vi "Com_SECS Equipment _Data Message Tree.vi"(8 "error in":errorcluster, 10 "SECS Packet":T1, 11 "Tree Refnum":refnum<vi>) -> (0 "error out":errorcluster)   [LabVIEW 2016]
uses:
  Data Def/Com_SECS Equipment _SECS Packet.ctl
  Data Def/Com_SECS Equipment _Message Type.ctl
  Data Def/Com_SECS Equipment _Protocol Type.ctl
  Data Def/Com_SECS Equipment _Stream Type.ctl
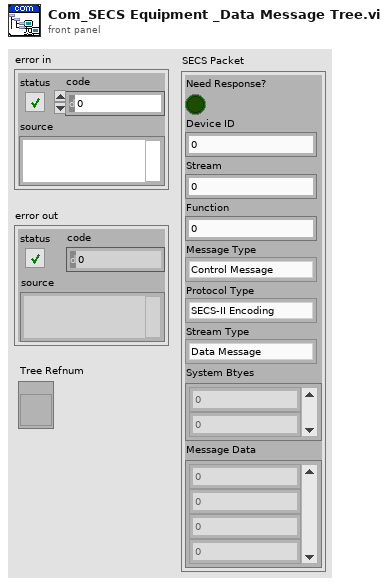
[diagram p1: front panel]
types:
  T1 = typedef "Com_SECS Equipment _SECS Packet.ctl" = cluster{"Need Response?":bool, "Device ID":u16, "Stream":u8, "Function":u8, "Message Type":T2, "Protocol Type":T3, "Stream Type":T4, "System Btyes":u8[], "Message Data":u8[]}
  T2 = typedef "Com_SECS Equipment _Message Type.ctl" = enum16{"Control Message", "Data Message"}
  T3 = typedef "Com_SECS Equipment _Protocol Type.ctl" = enum16{"SECS-II Encoding", "Reserved"}
  T4 = typedef "Com_SECS Equipment _Stream Type.ctl" = enum16{"Data Message", "Select.req", "Select.rsp", "Deselect.req", "Deselect.rsp", "Linktest.req", "Linktest.rsp", "Reject.req", "Separate.req", "Reserve"}
  T5 = typedef "Com_SECS Equipment _Message Data.ctl" = cluster{"Index":i32, "Data Item Format":T6, "Format Code":T7, "Parent Index":i32, "Child Index":i32[], "Data":variant}
  T6 = typedef "Com_SECS Equipment _Data Item Format.ctl" = enum16{"Data Type", "Value"}
  T7 = typedef "Com_SECS Equipment _Format Code.ctl" = enum16{"L", "A", "B", "Boolean", "J", "I1", "I2", "I4", "I8", "U1", "U2", "U4", "U8", "F4", "F8", "Char"}
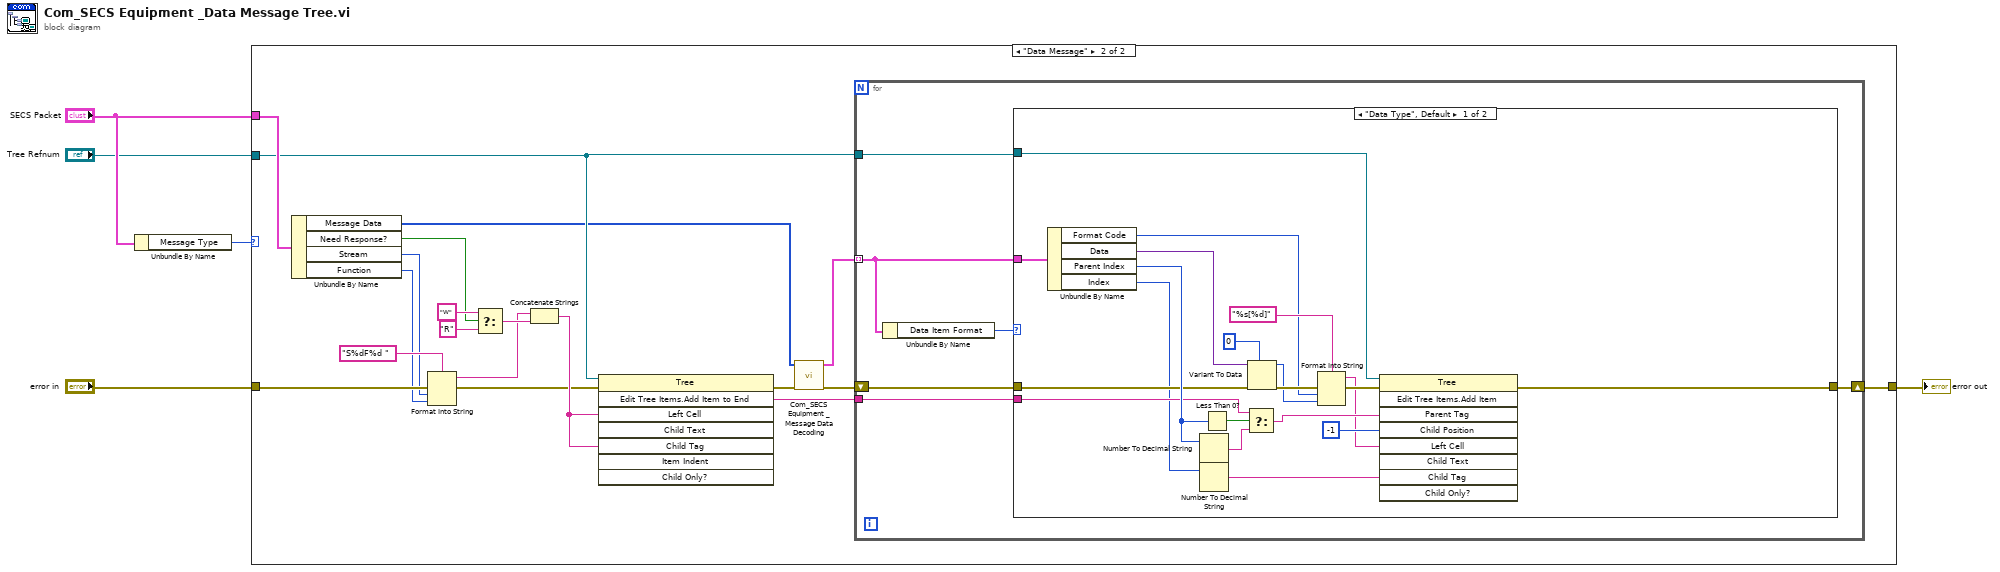
[diagram p0: block diagram]
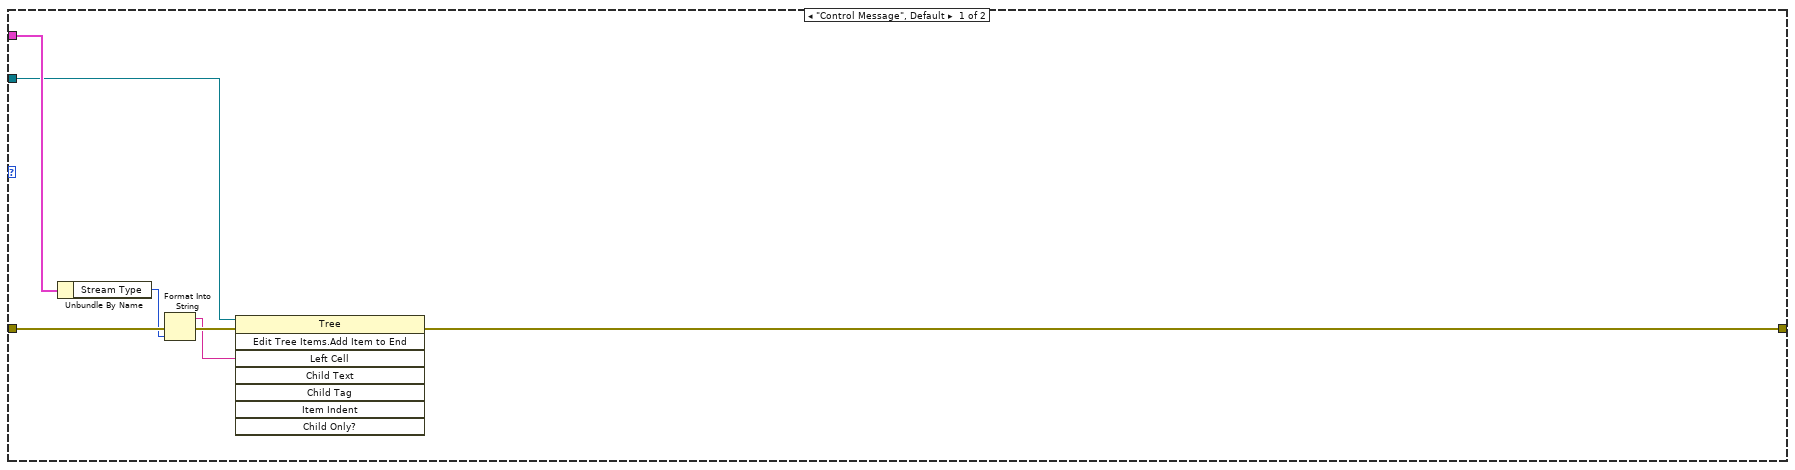
[diagram p2: hidden frame]
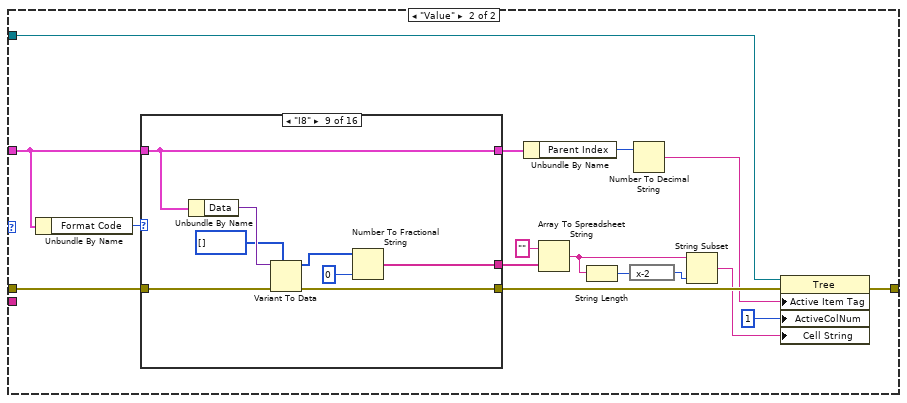
[diagram p3: hidden frame]
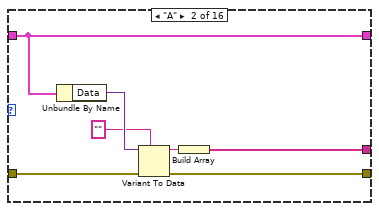
[diagram p5: hidden frame]
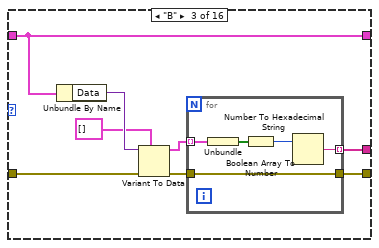
[diagram p6: hidden frame]
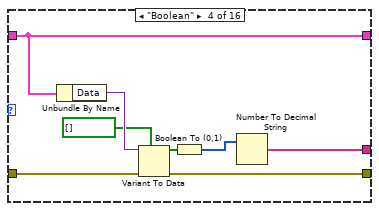
[diagram p7: hidden frame]
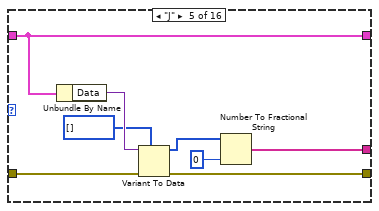
[diagram p8: hidden frame]
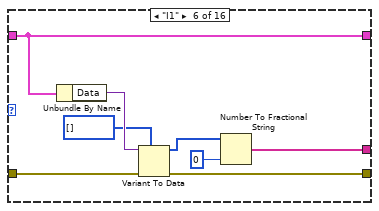
[diagram p9: hidden frame]
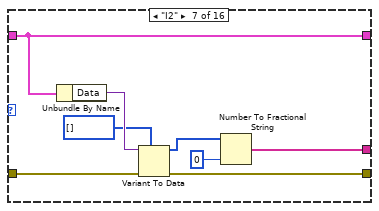
[diagram p10: hidden frame]
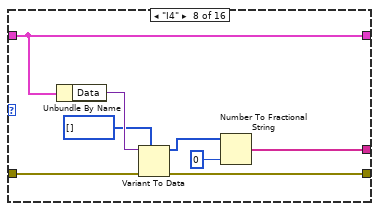
[diagram p11: hidden frame]
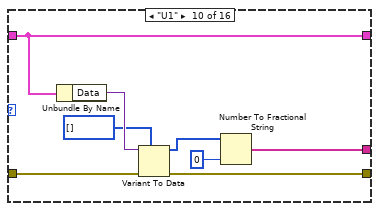
[diagram p12: hidden frame]
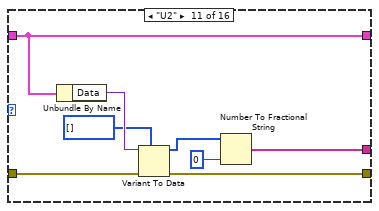
[diagram p13: hidden frame]
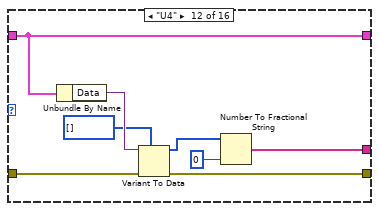
[diagram p14: hidden frame]
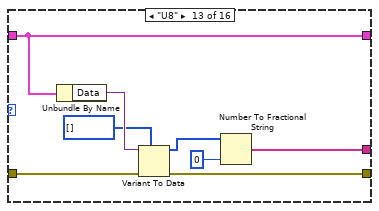
[diagram p15: hidden frame]
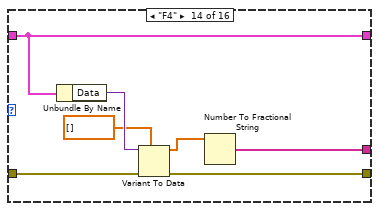
[diagram p16: hidden frame]
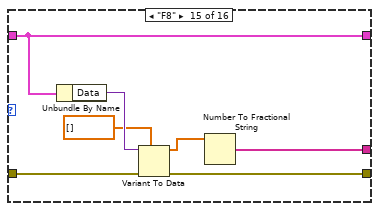
[diagram p17: hidden frame]
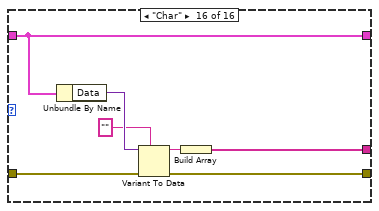
[diagram p18: hidden frame]
diagram:
  n1 = Unbundle By Name("SECS Packet") -> ("Message Type"=w5:T2)
  n2 = case shown="\"Data Message\"" w5 {
    tunnel: "error in" -> [w11 w23]
    tunnel: "SECS Packet" -> [w12 w31]
    tunnel: "Tree Refnum" -> [w8 w16]
    tunnel: [w6 w14] -> w1
    frame "Control Message", Default {
      n3 = Unbundle By Name(w12) -> ("Stream Type"=w10:T4)
      n4 = Format Into String(error in=w11, w10) -> (resulting string=w7:string, error out=w9:errorcluster)  [unwired: 2 in]
      n5 = invoke on="Invoke Node" class="Tree" method="Edit Tree Items.Add Item to End"(reference=w8, error in=w9, "Left Cell"=w7) -> (error out=w6:errorcluster)  [unwired: 5 in, 7 out]
    }
    frame "Data Message" {
      n6 = Unbundle By Name(w31) -> ("Message Data"=w13:u8[], "Need Response?"=w20:bool, "Stream"=w21:u8, "Function"=w22:u8)
      n7 = Format Into String(format string="S%dF%d ", error in=w23, w21, w22) -> (resulting string=w27:string, error out=w29:errorcluster)  [unwired: 1 in]
      n8 = Select(t="W", s=w20, f="R") -> (s? t:f=w28:string)
      n9 = Concatenate Strings(w27, w28) -> (w30:string)
      n10 = invoke on="Invoke Node" class="Tree" method="Edit Tree Items.Add Item to End"(reference=w16, error in=w29, "Left Cell"=w30, "Child Tag"=w30) -> (error out=w19:errorcluster, "Edit Tree Items:Add Item to End"=w17:string)  [unwired: 4 in, 6 out]
      n11 = call "Com_SECS Equipment _Message Data Decoding.vi"("error in"=w19, "Message Data In"=w13) -> ("error out"=w18:errorcluster, "Message Data Out"=w15:T5[])  [unwired: 7 in, 1 out]
      n12 = for {
        tunnel: w15 -> [w36] mode=indexing
        tunnel: w17 -> [w34]
        shift-right: [w33] -> w14
        shift-left: w18 -> [w35]
        tunnel: w16 -> [w32]
        n13 = Unbundle By Name(w36) -> ("Data Item Format"=w37:T6)
        n14 = case shown="\"Data Type\", Default" w37 {
          tunnel: w36 -> [w57 w71]
          tunnel: w35 -> [w51 w72]
          tunnel: w34 -> [w42 _]
          tunnel: [w39 w59] -> w33
          tunnel: w32 -> [w38 w58]
          frame "Data Type", Default {
            n15 = Unbundle By Name(w57) -> ("Format Code"=w46:T7, "Data"=w49:variant, "Parent Index"=w55:i32, "Index"=w41:i32)
            n16 = Number To Decimal String(number=w55) -> (decimal integer string=w43:string)  [unwired: 1 in]
            n17 = Number To Decimal String(number=w41) -> (decimal integer string=w40:string)  [unwired: 1 in]
            n18 = Less Than 0?(x=w55) -> (x < 0?=w56:bool)
            n19 = Select(t=w42, s=w56, f=w43) -> (s? t:f=w54:string)
            n20 = Variant To Data(error in=w51, type=u32 0, Variant=w49) -> (data=w47:u32, error out=w50:errorcluster)
            n21 = Format Into String(format string="%s[%d]", error in=w50, w46, w47) -> (resulting string=w44:string, error out=w45:errorcluster)  [unwired: 1 in]
            n22 = invoke on="Invoke Node" class="Tree" method="Edit Tree Items.Add Item"(reference=w38, error in=w45, "Parent Tag"=w54, "Child Position"=-1, "Left Cell"=w44, "Child Tag"=w40) -> (error out=w39:errorcluster)  [unwired: 3 in, 8 out]
          }
          frame "Value" {
            n23 = Unbundle By Name(w71) -> ("Format Code"=w73:T7)
            n24 = case shown="\"I8\"" w73 {
              tunnel: w72 -> [w75 w82 w90 w103 w111 w119 w127 w135 w143 w151 w159 w167 w175 w182 w189 w196]
              tunnel: w71 -> [w74 w78 w88 w101 w109 w117 w125 w133 w141 w149 w157 w165 w173 w180 w187 w194]
              tunnel: [w75 w79 w84 w99 w108 w116 w124 w132 w140 w148 w156 w164 w172 w179 w186 w193] -> w65
              tunnel: [w74 w78 w88 w101 w109 w117 w125 w133 w141 w149 w157 w165 w173 w180 w187 w194] -> w64
              tunnel: [_ w76 w83 w98 w107 w115 w123 w131 w139 w147 w155 w163 w171 w178 w185 w190] -> w70
              frame "L", Default {
              }
              frame "A" {
                n25 = Unbundle By Name(w78) -> ("Data"=w81:variant)
                n26 = Variant To Data(error in=w82, type="", Variant=w81) -> (data=w77:string, error out=w79:errorcluster)
                n27 = Build Array(w77) -> (w76:string[])
              }
              frame "B" {
                n28 = Unbundle By Name(w88) -> ("Data"=w89:variant)
                n29 = Variant To Data(error in=w90, type=cluster{"Boolean array":bool[]}[] [], Variant=w89) -> (data=w85:cluster{"Boolean array":bool[]}[], error out=w86:errorcluster)
                n30 = for {
                  tunnel: w86 -> [w93]
                  tunnel: w85 -> [w95] mode=indexing
                  tunnel: [w93] -> w84
                  tunnel: [w91] -> w83 mode=indexing
                  n31 = Unbundle(w95) -> ("Boolean array"=w94:bool[])
                  n32 = Boolean Array To Number(Boolean array=w94) -> (number=w92:u32)
                  n33 = Number To Hexadecimal String(2:w92) -> (0:w91:string)  [unwired: 1 in]
                }
              }
              frame "Boolean" {
                n34 = Unbundle By Name(w101) -> ("Data"=w102:variant)
                n35 = Variant To Data(error in=w103, type=bool[] [], Variant=w102) -> (data=w100:bool[], error out=w99:errorcluster)
                n36 = Boolean To (0,1)(Boolean=w100) -> (0, 1=w96:i16[])
                n37 = Number To Decimal String(number=w96) -> (decimal integer string=w98:string[])  [unwired: 1 in]
              }
              frame "J" {
                n38 = Unbundle By Name(w109) -> ("Data"=w110:variant)
                n39 = Variant To Data(error in=w111, type=u8[] [], Variant=w110) -> (data=w105:u8[], error out=w108:errorcluster)
                n40 = Number To Fractional String(number=w105, precision (6)=i16 0) -> (F-format string=w107:string[])  [unwired: 2 in]
              }
              frame "I1" {
                n41 = Unbundle By Name(w117) -> ("Data"=w118:variant)
                n42 = Variant To Data(error in=w119, type=i8[] [], Variant=w118) -> (data=w113:i8[], error out=w116:errorcluster)
                n43 = Number To Fractional String(number=w113, precision (6)=i16 0) -> (F-format string=w115:string[])  [unwired: 2 in]
              }
              frame "I2" {
                n44 = Unbundle By Name(w125) -> ("Data"=w126:variant)
                n45 = Variant To Data(error in=w127, type=i16[] [], Variant=w126) -> (data=w121:i16[], error out=w124:errorcluster)
                n46 = Number To Fractional String(number=w121, precision (6)=i16 0) -> (F-format string=w123:string[])  [unwired: 2 in]
              }
              frame "I4" {
                n47 = Unbundle By Name(w133) -> ("Data"=w134:variant)
                n48 = Variant To Data(error in=w135, type=i32[] [], Variant=w134) -> (data=w129:i32[], error out=w132:errorcluster)
                n49 = Number To Fractional String(number=w129, precision (6)=i16 0) -> (F-format string=w131:string[])  [unwired: 2 in]
              }
              frame "I8" {
                n50 = Unbundle By Name(w141) -> ("Data"=w142:variant)
                n51 = Variant To Data(error in=w143, type=i64[] [], Variant=w142) -> (data=w137:i64[], error out=w140:errorcluster)
                n52 = Number To Fractional String(number=w137, precision (6)=i16 0) -> (F-format string=w139:string[])  [unwired: 2 in]
              }
              frame "U1" {
                n53 = Unbundle By Name(w149) -> ("Data"=w150:variant)
                n54 = Variant To Data(error in=w151, type=u8[] [], Variant=w150) -> (data=w145:u8[], error out=w148:errorcluster)
                n55 = Number To Fractional String(number=w145, precision (6)=i16 0) -> (F-format string=w147:string[])  [unwired: 2 in]
              }
              frame "U2" {
                n56 = Unbundle By Name(w157) -> ("Data"=w158:variant)
                n57 = Variant To Data(error in=w159, type=u16[] [], Variant=w158) -> (data=w153:u16[], error out=w156:errorcluster)
                n58 = Number To Fractional String(number=w153, precision (6)=i16 0) -> (F-format string=w155:string[])  [unwired: 2 in]
              }
              frame "U4" {
                n59 = Unbundle By Name(w165) -> ("Data"=w166:variant)
                n60 = Variant To Data(error in=w167, type=u32[] [], Variant=w166) -> (data=w161:u32[], error out=w164:errorcluster)
                n61 = Number To Fractional String(number=w161, precision (6)=i16 0) -> (F-format string=w163:string[])  [unwired: 2 in]
              }
              frame "U8" {
                n62 = Unbundle By Name(w173) -> ("Data"=w174:variant)
                n63 = Variant To Data(error in=w175, type=u64[] [], Variant=w174) -> (data=w169:u64[], error out=w172:errorcluster)
                n64 = Number To Fractional String(number=w169, precision (6)=i16 0) -> (F-format string=w171:string[])  [unwired: 2 in]
              }
              frame "F4" {
                n65 = Unbundle By Name(w180) -> ("Data"=w181:variant)
                n66 = Variant To Data(error in=w182, type=sgl[] [], Variant=w181) -> (data=w176:sgl[], error out=w179:errorcluster)
                n67 = Number To Fractional String(number=w176) -> (F-format string=w178:string[])  [unwired: 3 in]
              }
              frame "F8" {
                n68 = Unbundle By Name(w187) -> ("Data"=w188:variant)
                n69 = Variant To Data(error in=w189, type=dbl[] [], Variant=w188) -> (data=w183:dbl[], error out=w186:errorcluster)
                n70 = Number To Fractional String(number=w183) -> (F-format string=w185:string[])  [unwired: 3 in]
              }
              frame "Char" {
                n71 = Unbundle By Name(w194) -> ("Data"=w195:variant)
                n72 = Variant To Data(error in=w196, type="", Variant=w195) -> (data=w191:string, error out=w193:errorcluster)
                n73 = Build Array(w191) -> (w190:string[])
              }
            }
            n74 = Unbundle By Name(w64) -> ("Parent Index"=w63:i32)
            n75 = Array To Spreadsheet String(array=w70, 3:"" ("format string")) -> (spreadsheet string=w68:string)  [unwired: 1 in]
            n76 = String Length(string=w68) -> (length=w67:i32)
            n77 = expression code="x-2"(w67) -> (w66:i32)
            n78 = Number To Decimal String(number=w63) -> (decimal integer string=w62:string)  [unwired: 1 in]
            n79 = String Subset(string=w68, length (rest)=w66) -> (substring=w60:string)  [unwired: 1 in]
            n80 = property on="Property Node" class="Tree"(reference=w58, error in=w65, "Active Item Tag"=w62, "ActiveColNum"=1 ("Active Cell:Active Column Number"), "Cell String"=w60) -> (error out=w59:errorcluster)  [unwired: 1 out]
          }
        }
      }
    }
  }
  "error out" <- w1
